vi "Begin.vi"(8 "error in (no error)":errorcluster, 9 "Intake Right Channel":T1=enum."PWM 1", 10 "Intake Left Channel":T1, 11 "Cargo Concrete in":refnum<class "Cargo Concrete.lvclass">) -> (0 "error out":errorcluster, 3 "Cargo Concrete out":refnum<class "Cargo Concrete.lvclass">)   [LabVIEW 2018, in "Cargo.lvlib" / "Cargo Concrete.lvclass"]
uses:
  Cargo Concrete.lvclass
  <vilib>/Rock Robotics/SystemInterfaces/DIO/FPGA_DIOPWMChannel.ctl
  Cargo Concrete.lvclass/Cargo Concrete.ctl
  <vilib>/Rock Robotics/WPI/MotorControl/WPI_MotorControlOpen VictorSP.vi
  Cargo.lvclass
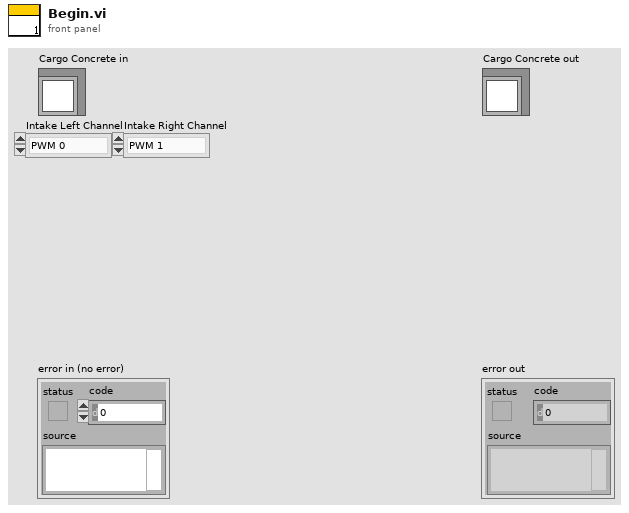
[diagram p1: front panel]
types:
  T1 = typedef "FPGA_DIOPWMChannel.ctl" = enum8{"PWM 0", "PWM 1", "PWM 2", "PWM 3", "PWM 4", "PWM 5", "PWM 6", "PWM 7", "PWM 8", "PWM 9", "PWM MXP 0", "PWM MXP 1", "PWM MXP 2", "PWM MXP 3", "PWM MXP 4", "PWM MXP 5", "PWM MXP 6", "PWM MXP 7", "PWM MXP 8", "PWM MXP 9", "Invalid"}
  T2 = typedef "WPI_MotorControlDeviceRef.ctl" = cluster{"DeviceStatus":errorcluster, "Type":T3, "PWM":cluster{"PWM Channel":T1, "DeadBand":T4}, "CAN":cluster{"Device Number":u8, "SetOutput VI Ref":variant, "GetOutput VI Ref":variant, "Enable VI Ref":variant, "Disable VI Ref":variant, "Data":variant}, "Invert":bool, "DIO PWM":cluster{"PWM \"Enable\" Channel":T1, "DIOChannel":T5, "PWM Rate":dbl}}
  T3 = typedef "WPI_MotorControlType.ctl" = enum16{"PWM", "CAN", "DIO PWM"}
  T4 = typedef "WPI_PWMDeadband.ctl" = cluster{"Name":string, "maxPositivePwm":i32, "minPositivePwm":i32, "centerPwm":i32, "maxNegativePwm":i32, "minNegativePwm":i32, "angularRange":u16}
  T5 = typedef "FPGA_DIOChannel.ctl" = enum8{"DIO 0", "DIO 1", "DIO 2", "DIO 3", "DIO 4", "DIO 5", "DIO 6", "DIO 7", "DIO 8", "DIO 9", "DIO MXP 0", "DIO MXP 1", "DIO MXP 2", "DIO MXP 3", "DIO MXP 4", "DIO MXP 5", "DIO MXP 6", "DIO MXP 7", "DIO MXP 8", "DIO MXP 9", "DIO MXP 10", "DIO MXP 11", "DIO MXP 12", "DIO MXP 13", "DIO MXP 14", "DIO MXP 15", "SPI Port CS1", "SPI Port CS2", "SPI Port CS3", "SPI Port MISO", "SPI Port MOSI", "Invalid"}
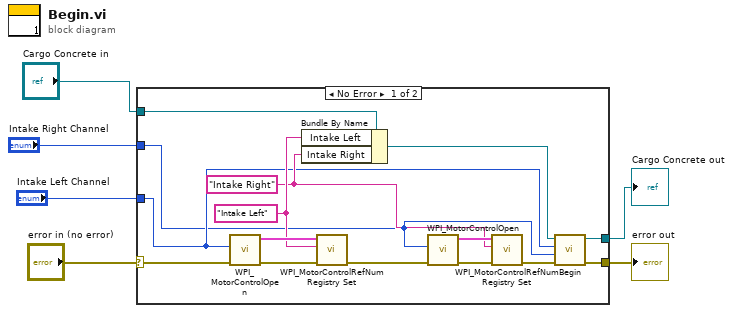
[diagram p0: block diagram]
diagram:
  n1 = case shown="No Error" "error in (no error)" {
    selector: "error in (no error)" -> [w19 w23]
    tunnel: [w21 w23] -> w6
    tunnel: [w20 w22] -> w5
    tunnel: "Intake Left Channel" -> [w9 _]
    tunnel: "Intake Right Channel" -> [w8 _]
    tunnel: "Cargo Concrete in" -> [w7 w22]
    frame No Error {
      w10 = "Intake Right" ("refnum name")
      w11 = "Intake Left" ("refnum name")
      n2 = call-poly <vilib>:"WPI_MotorControlOpen.vi"("error in (no error)"=w19, "PWM Channel"=w9) -> ("error out"=w15:errorcluster, "MotorControlDeviceRef"=w16:T2)  [unwired: 8 in]
      n3 = Bundle By Name(cluster=w7, "Intake Left"=w11, "Intake Right"=w10) -> (w17:refnum<class "Cargo Concrete.lvclass">)
      n4 = call <vilib>:"WPI_MotorControlRefNum Registry Set.vi"("error in (no error)"=w15, "refnum name"=w11, "MotorControlDevRef"=w16) -> ("error out"=w12:errorcluster)  [unwired: 7 in, 1 out]
      n5 = call-poly <vilib>:"WPI_MotorControlOpen.vi"("error in (no error)"=w12, "PWM Channel"=w8) -> ("error out"=w13:errorcluster, "MotorControlDeviceRef"=w14:T2)  [unwired: 8 in]
      n6 = call <vilib>:"WPI_MotorControlRefNum Registry Set.vi"("error in (no error)"=w13, "refnum name"=w10, "MotorControlDevRef"=w14) -> ("error out"=w18:errorcluster)  [unwired: 7 in, 1 out]
      n7 = call-parent "Begin.vi"("error in (no error)"=w18, "Intake Right Channel"=w8, "Intake Left Channel"=w9, "Cargo in"=w17) -> ("error out"=w21:errorcluster, "Cargo out"=w20:refnum<class "Cargo Concrete.lvclass">)  [unwired: 6 in]
    }
    frame Error {
    }
  }
  "error out" <- w6
  "Cargo Concrete out" <- w5
